vi "_Read CSM Status Content.vi"(8 "error in (no error)":errorcluster, 11 "CSM-Helper in":refnum<class "CSM-Helper.lvclass">) -> (0 "error out":errorcluster, 2 "Array":string[](array[string]), 3 "CSM-Helper out":refnum<class "CSM-Helper.lvclass">)   [LabVIEW 2017, in "CSM-Helper API with lvcsm Support.lvlib"]
uses:
  CSM-Helper API with lvcsm Support.lvlib
  CSM-Helper.lvclass
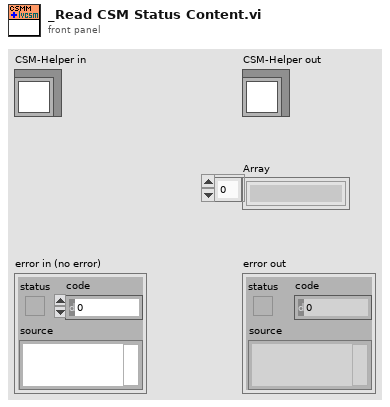
[diagram p1: front panel]
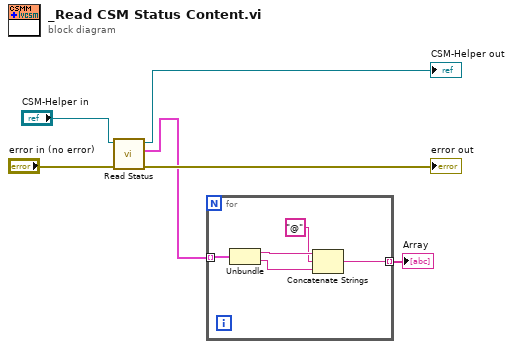
[diagram p0: block diagram]
diagram:
  n1 = call "Read Status.vi"("error in (no error)"="error in (no error)", "CSM-Helper in"="CSM-Helper in") -> ("error out"=→"error out":errorcluster, "Array 3"=w2:cluster{"Status":string, "InState":string}[], "CSM-Helper out"=→"CSM-Helper out":refnum<class "CSM-Helper.lvclass">)  [unwired: 7 in]
  n2 = for {
    tunnel: w2 -> [w11] mode=indexing
    tunnel: [w7] -> w1 mode=indexing
    n3 = Unbundle(w11) -> ("Status"=w10:string, "InState"=w9:string)
    n4 = Concatenate Strings(w10, "@" ("string"), w9) -> (w7:string)
  }
  "Array" <- w1
